vi "Populate Control.vi"() -> ()   [LabVIEW 2013]
uses:
  C:/Program Files/Princeton Instruments/LightField/PrincetonInstruments.LightFieldAddInSupportServices.dll
  Program Files/Princeton Instruments/LightField/PrincetonInstruments.LightFieldAddInSupportServices.dll
  lightfield-automation-labview/LightField Automation.lvclass
panel:
  in  "Experiment Name":string
  in  "stop":bool
  in  "ADC Quality (Ring Control I32 Representation)":i32(ring)
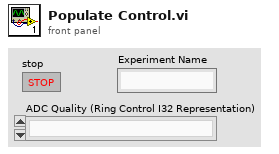
[diagram p1: front panel]
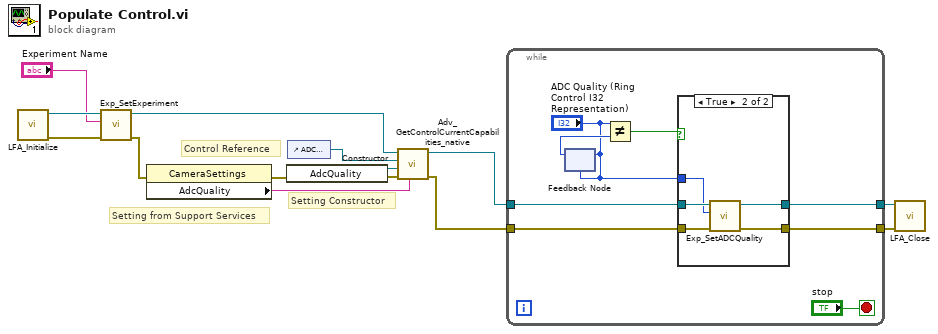
[diagram p0: block diagram]
diagram:
  # "Control Reference"
  # "Setting Constructor"
  # "Setting from Support Services"
  n1 = call "LFA_Initialize.vi"() -> ("error out"=w6:errorcluster, "LightField Automation out"=w7:refnum<class "LightField Automation.lvclass">)  [unwired: 10 in]
  n2 = call "Exp_SetExperiment.vi"("error in (no error)"=w6, "ExperimentName"="Experiment Name", "LightField Automation in"=w7) -> ("error out"=w3:errorcluster, "LightField Automation out"=w4:refnum<class "LightField Automation.lvclass">)  [unwired: 7 in]
  n3 = property class="CameraSettings"(error in=w3) -> (error out=w10:errorcluster, "AdcQuality"=w12:string)  [unwired: 1 in, 1 out]
  n4 = constructor class="AdcQuality"(error in=w10) -> (reference out=w14:refnum<k24>, error out=w11:errorcluster)  [unwired: 2 in, 1 out]
  n5 = control-ref of="ADC Quality (Ring Control I32 Representation)"() -> (w13:refnum<vi>)
  n6 = call "Adv_GetControlCurrentCapabilities_native.vi"("LightField Setting"=w12, "error in (no error)"=w11, "Enum Class"=w14, "Control"=w13, "LightField Automation in"=w4) -> ("error out"=w8:errorcluster, "LightField Automation out"=w9:refnum<class "LightField Automation.lvclass">)  [unwired: 5 in]
  n7 = while {
    tunnel: w9 -> [w19]
    tunnel: w8 -> [w18]
    tunnel: [w16] -> w1
    tunnel: [w15] -> w2
    stop <- "stop" stop-if-true
    n8 = feedback-in #1("ADC Quality (Ring Control I32 Representation)") -> ()
    n9 = feedback #1("ADC Quality (Ring Control I32 Representation)") -> (w21:i32)
    n10 = Not Equal?(x="ADC Quality (Ring Control I32 Representation)", y=w21) -> (x != y?=w20:bool)
    n11 = case shown="True" w20 {
      tunnel: w19 -> [w24 w29]
      tunnel: w18 -> [w23 w28]
      tunnel: "ADC Quality (Ring Control I32 Representation)" -> [_ w27]
      tunnel: [w24 w26] -> w16
      tunnel: [w23 w25] -> w15
      frame False {
      }
      frame True {
        n12 = call "Exp_SetADCQuality.vi"("error in (no error)"=w28, "ADCQuality"=w27, "LightField Automation in"=w29) -> ("error out"=w25:errorcluster, "LightField Automation out"=w26:refnum<class "LightField Automation.lvclass">)  [unwired: 7 in]
      }
    }
  }
  n13 = call "LFA_Close.vi"("error in (no error)"=w2, "LightField Automation in"=w1) -> ()  [unwired: 8 in, 2 out]
